vi "mes~Login Dialog.vi"(8 "错误输入（无错误）":errorcluster) -> (0 "错误常量":errorcluster, 2 "Success?":bool)   [LabVIEW 2015]
uses:
  <vilib>/Utility/miscctls.llb/LVPointTypeDef.ctl
  Global.vi
panel:
  in  "登录":bool
  in  "Password":string caption="密   码:"
  in  "UserName":string caption="用户名:"
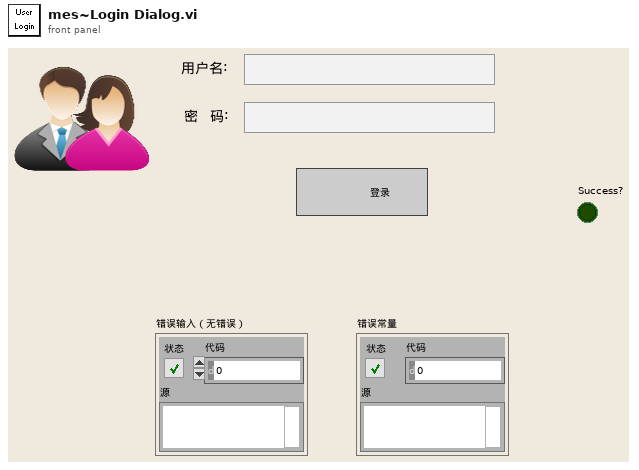
[diagram p1: front panel]
types:
  T1 = typedef "LVPointTypeDef.ctl" = cluster{"Horizontal":i16, "Vertical":i16}
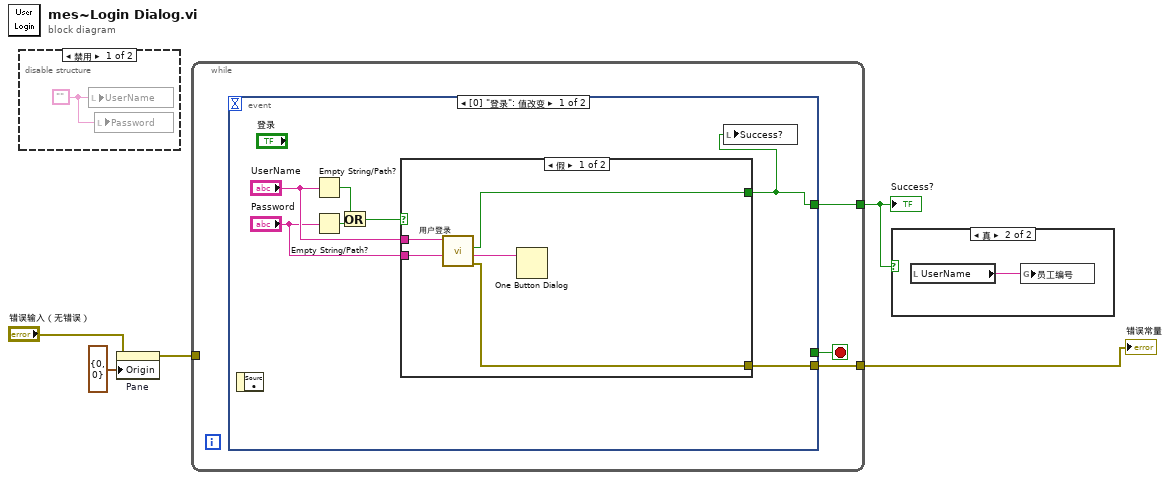
[diagram p0: block diagram]
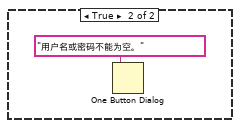
[diagram p4: hidden frame]
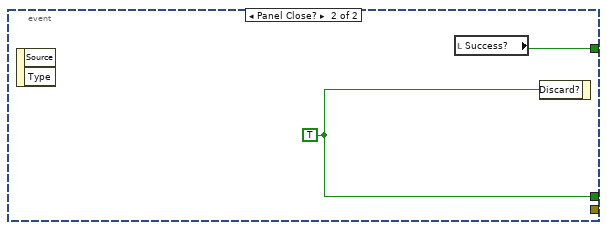
[diagram p5: hidden frame]
diagram:
  n1 = disable-structure shown="禁用" {
    frame Disabled {
      w6 = ""
      n2 = local write "UserName"(w6) -> ()
      n3 = local write "Password"(w6) -> ()
    }
    frame Enabled {
    }
  }
  n4 = property on="Pane" class="Pane"(error in="错误输入（无错误）", "Origin"=T1 {"Horizontal"=0, "Vertical"=0}) -> (error out=w4:errorcluster)  [unwired: 1 in, 1 out]
  n5 = while {
    tunnel: [w8] -> w3
    tunnel: w4 -> [_]
    tunnel: [w7] -> w1
    stop <- w9 stop-if-true
    n6 = event shown="[0] \"登录\": 值改变" {
      selector: _ -> [_ _]
      dyn-events: _ -> [_ _]
      timeout: _ -> [_ _]
      tunnel: [_ w24] -> w9
      tunnel: [w11 w23] -> w8
      tunnel: [w10 _] -> w7
      event "登录": Value Change {
        n7 = event-data() -> ()  [unwired: 1 in, 1 out]
        n8 = Empty String/Path?(string/path="UserName") -> (empty?=w15:bool)
        n9 = Empty String/Path?(string/path="Password") -> (empty?=w16:bool)
        n10 = Or(x=w15, y=w16) -> (x .or. y?=w14:bool)
        n11 = case shown="假" w14 {
          tunnel: "UserName" -> [w21 _]
          tunnel: "Password" -> [w20 _]
          tunnel: [w19 _] -> w11
          tunnel: [w18 _] -> w10
          frame False {
            n12 = call "用户登录.vi"("Password"=w20, "UserName"=w21) -> ("error out"=w18:errorcluster, "ErrorMessage"=w17:string, "登录成功"=w19:bool)  [unwired: 7 in]
            n13 = One Button Dialog(message=w17) -> ()  [unwired: 1 in, 1 out]
          }
          frame True {
            n14 = One Button Dialog(message="用户名或密码不能为空。") -> ()  [unwired: 1 in, 1 out]
          }
        }
        n15 = local write "Success?"(w11) -> ()
      }
      event Panel Close? {
        w24 = TRUE
        n16 = event-data() -> ()  [unwired: 1 in, 2 out]
        n17 = local read "Success?"() -> (w23:bool)
        n18 = event-data("Discard?"=w24) -> ()  [unwired: 1 in, 1 out]
      }
    }
  }
  "Success?" <- w3
  "错误常量" <- w1
  n19 = case shown="真" w3 {
    frame False {
    }
    frame True {
      n20 = local read "UserName"() -> (w25:string)
      n21 = global write "Global.vi" "员工编号"(w25) -> ()
    }
  }
